vi "XY Graph Clear Event.vi"(8 "Error In":errorcluster, 11 "XYGraph Ref":T1) -> (0 "Error Out":errorcluster, 1 "Message":string, 3 "Graph Caption":string)   [LabVIEW 2019, in "XY Graph Add-Ons.lvlib"]
uses:
  XY Graph Add-Ons.lvlib
  XY Graph Refnum.ctl
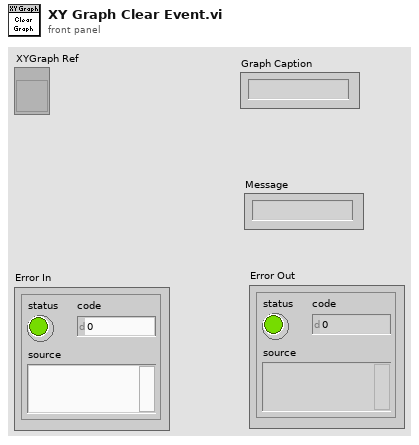
[diagram p1: front panel]
types:
  T1 = typedef "XY Graph Add-Ons.lvlib/XY Graph Refnum.ctl" = refnum<vi>
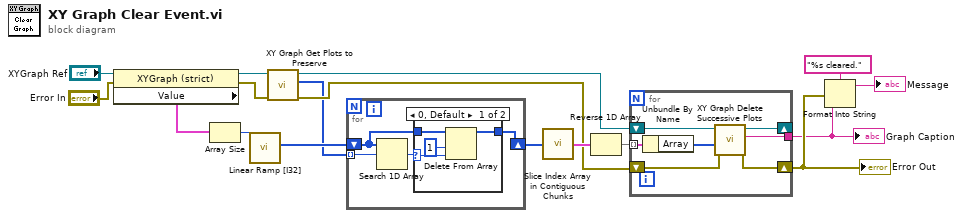
[diagram p0: block diagram]
diagram:
  n1 = property class="XYGraph (strict)"(reference="XYGraph Ref", error in="Error In") -> (reference out=w9:T1, error out=w7:errorcluster, "Value"=w10:cluster{"X Array":dbl[], "Y Array":dbl[]}[])
  n2 = Array Size(array=w10) -> (size(s)=w12:i32)
  n3 = call "Linear Ramp [I32].vi"("# Elements"=w12) -> ("Ramp"=w11:i32[])  [unwired: 8 in]
  n4 = call "XY Graph Get Plots to Preserve.vi"("Error In"=w7, "XYGraph in"=w9) -> ("Error Out"=w6:errorcluster, "Preserved Plots"=w5:i32[], "XYGraph out"=w8:T1)  [unwired: 6 in, 1 out]
  n5 = for {
    tunnel: w5 -> [w21] mode=indexing
    shift-right: [w18] -> w17
    shift-left: w11 -> [w19]
    n6 = Search 1D Array(1D array=w19, element=w21) -> (index of element=w20:i32)  [unwired: 1 in]
    n7 = case shown="0, Default" w20 {
      selector: w20 -> [w24 _]
      tunnel: w19 -> [w25 w26]
      tunnel: [w23 w26] -> w18
      frame 0, Default {
        n8 = Delete From Array(array=w25, length=1, index=w24) -> (array with subset deleted=w23:i32[])  [unwired: 1 out]
      }
      frame -1 {
      }
    }
  }
  n9 = call "Slice Index Array in Contiguous Chunks.vi"("Array in"=w17) -> ("Contiguous sub-Arrays"=w16:cluster{"Array":i32[]}[])  [unwired: 8 in]
  n10 = Reverse 1D Array(array=w16) -> (reversed array=w15:cluster{"Array":i32[]}[])
  n11 = for {
    tunnel: w15 -> [w33] mode=indexing
    shift-right: [w30] -> _
    shift-left: w8 -> [w31]
    tunnel: [w29] -> w3
    shift-right: [w27] -> w4
    shift-left: w6 -> [w28]
    n12 = Unbundle By Name(w33) -> ("Array"=w32:i32[])
    n13 = call "XY Graph Delete Successive Plots.vi"("Error In"=w28, "Plot Indices"=w32, "XYGraph Ref"=w31) -> ("Error Out"=w27:errorcluster, "Graph Caption"=w29:string, "XYGraph Ref"=w30:refnum<vi>)  [unwired: 5 in, 1 out]
  }
  "Error Out" <- w4
  "Graph Caption" <- w3
  n14 = Format Into String(format string="%s cleared.", error in=w4, w3) -> (resulting string=→"Message":string)  [unwired: 1 in, 1 out]
